vi "Page Test.vi"() -> ()   [LabVIEW 2018, in "Page.lvlib"]
uses:
  Page.lvlib
panel:
  out "Time":timestamp
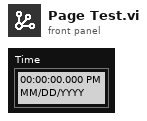
[diagram p1: front panel]
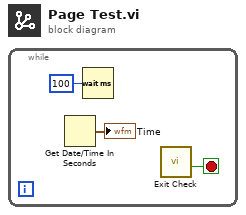
[diagram p0: block diagram]
diagram:
  n1 = while {
    stop <- w1 stop-if-true
    n2 = Get Date/Time In Seconds() -> (seconds since 1Jan1904=→"Time":timestamp)
    n3 = Wait (ms)(milliseconds to wait=u32 100) -> ()  [unwired: 1 out]
    n4 = call "Exit Check.vi"() -> ("Exit?"=w1:bool)  [unwired: 10 in, 1 out]
  }
